vi "Create UI_DSP_config.vi"(8 "error in (no error)":errorcluster, 10 "DSP.lvclass":refnum<class "DSP.lvclass">, 11 "UI_DSP_Config.lvclass":refnum<class "UI_DSP_Config.lvclass">) -> (0 "error out":errorcluster, 3 "output cluster":refnum<class "UI_DSP_Config.lvclass">)   [LabVIEW 2016, in "UI_DSP_Config.lvclass"]
uses:
  UI_DSP_Config.lvclass
  C:/Program Files (x86)/National Instruments/LabVIEW 2016/vi.lib/JKI/JKI SMO/SMO/SMO.lvclass
  DSP/DSP.lvclass
  UI_DSP_Config.lvclass/UI_DSP_Config.ctl
  <vilib>/JKI/JKI SMO/SMO/SMO.lvclass
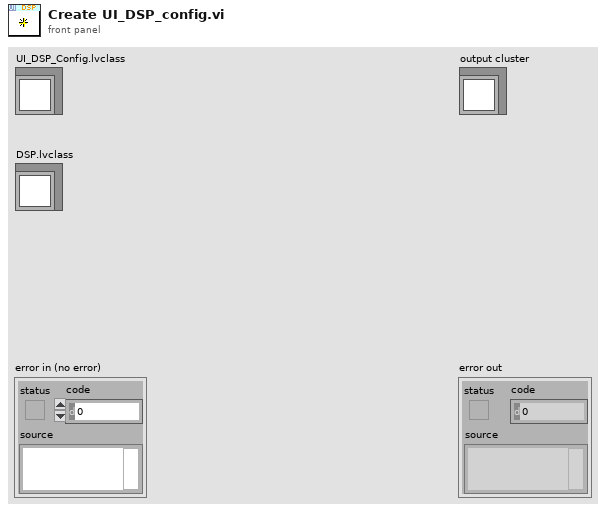
[diagram p1: front panel]
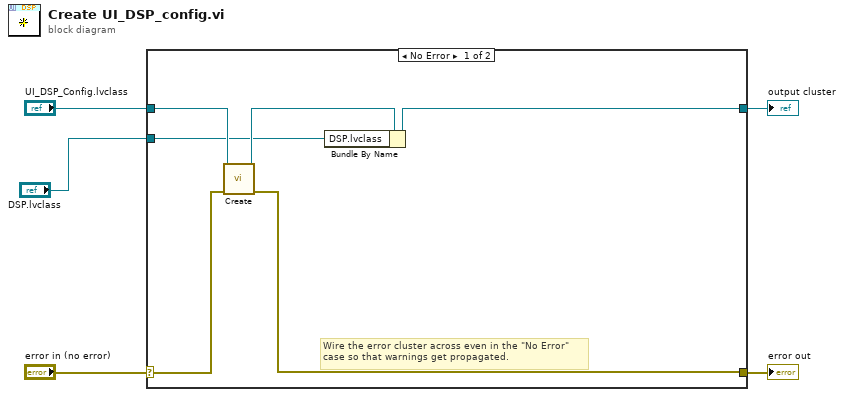
[diagram p0: block diagram]
diagram:
  n1 = case shown="No Error" "error in (no error)" {
    selector: "error in (no error)" -> [w10 w13]
    tunnel: [w9 w13] -> w4
    tunnel: "UI_DSP_Config.lvclass" -> [w8 w12]
    tunnel: [w11 w12] -> w2
    tunnel: "DSP.lvclass" -> [w6 _]
    frame No Error {
      # "Wire the error cluster across even in the \"No Error\"\ncase so that warnings get propagated."
      n2 = call <vilib>:"Create.vi"("error in (no error)"=w10, "SMO"=w8) -> ("error out"=w9:errorcluster, "SMO out"=w7:refnum<class "UI_DSP_Config.lvclass">)  [unwired: 7 in, 1 out]
      n3 = Bundle By Name(cluster=w7, "DSP.lvclass"=w6) -> (w11:refnum<class "UI_DSP_Config.lvclass">)
    }
    frame Error {
    }
  }
  "error out" <- w4
  "output cluster" <- w2
